vi "approach monitor.vi"() -> ()   [LabVIEW 2021]
uses:
  <userlib>/Nanonis Prog Interface V5/Nanonis Prog Interface.lvlib
panel:
  in  "Walker voltage (V)":dbl=220.0
  in  "stop":bool
  in  "Time between checks (ms)":i32=20000
  in  "Averages":i32=50
  in  "milliseconds to wait":u32=1000
  out "Delta":cluster{i32, sgl}[](graph)
  out "Capacitance":cluster{i32, sgl}[](graph)
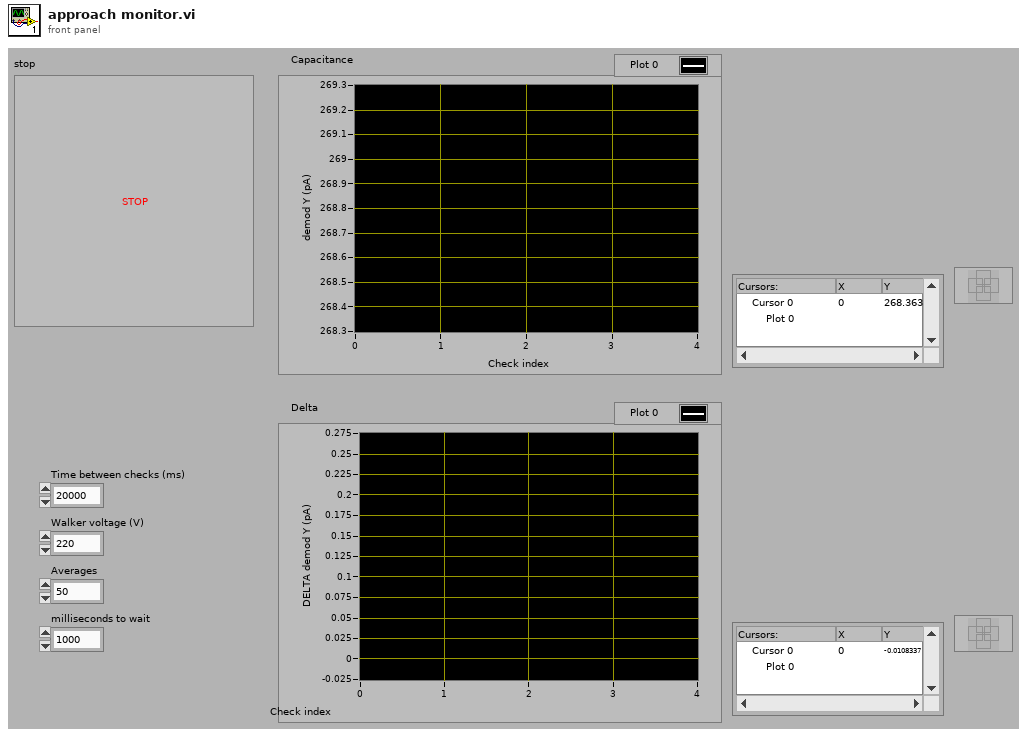
[diagram p1: front panel]
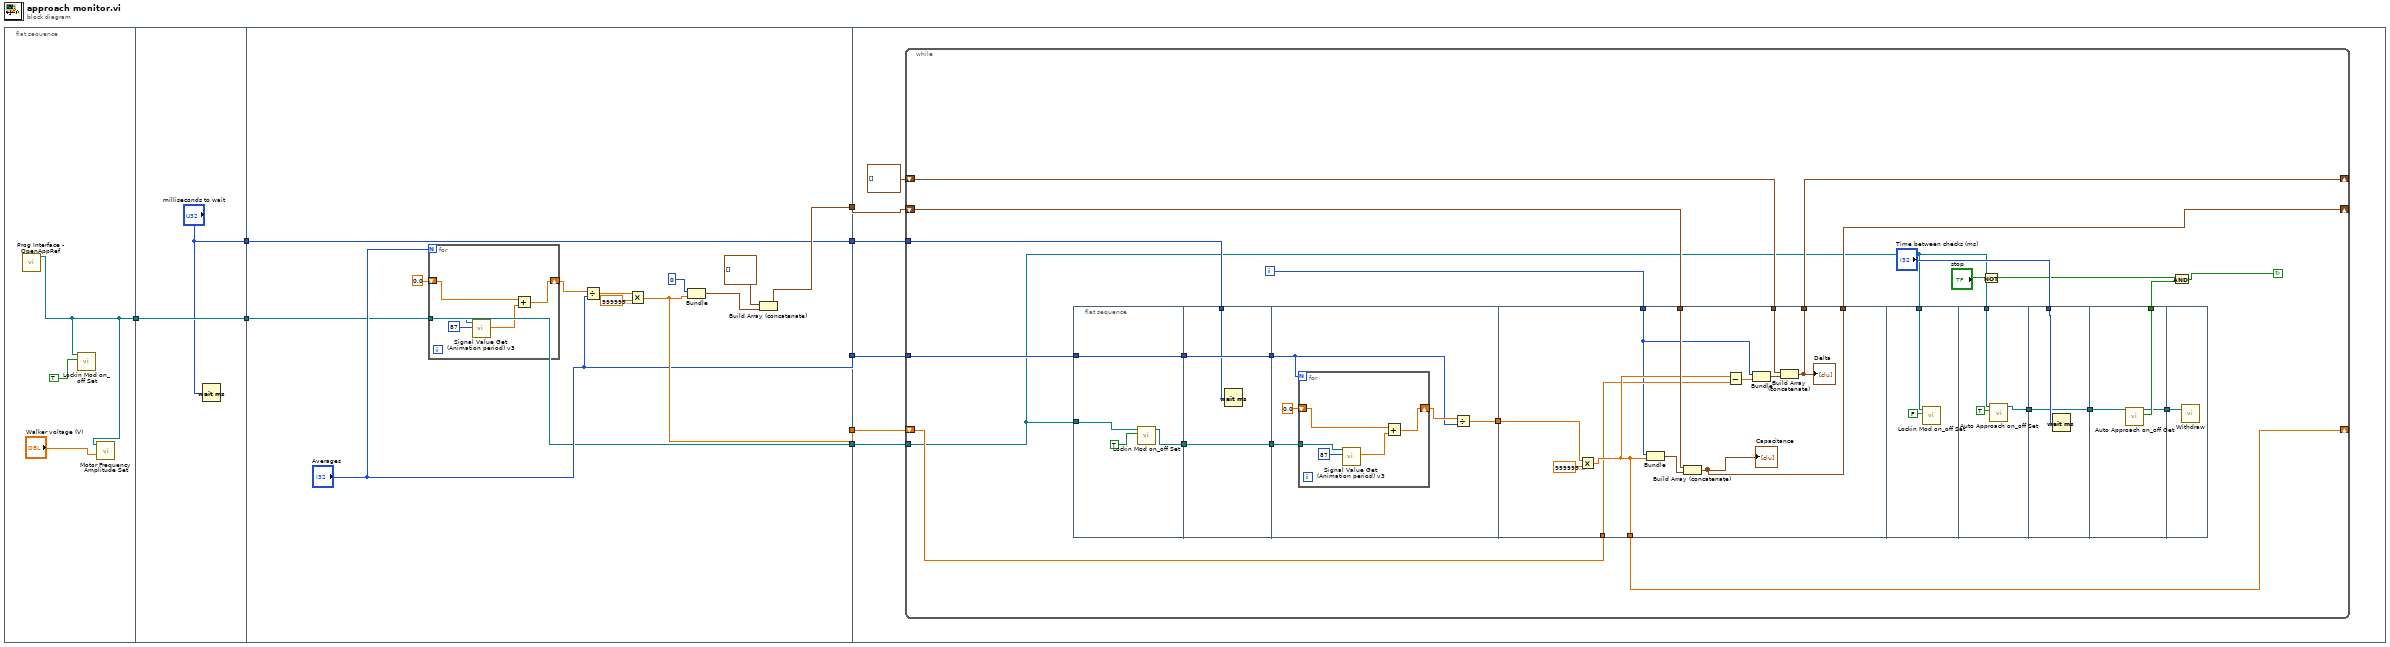
[diagram p0: block diagram]
diagram:
  n1 = flat-sequence {
    tunnel: [w9] -> w3
    tunnel: w3 -> [w13]
    tunnel: [w13] -> w2
    tunnel: ["milliseconds to wait"] -> w1
    tunnel: ["Averages"] -> w8
    tunnel: [w18] -> w7
    tunnel: [w21] -> w6
    tunnel: [w20] -> w5
    tunnel: w2 -> [w18]
    tunnel: [w17] -> w4
    tunnel: w1 -> [w17]
    tunnel: w8 -> [w36]
    tunnel: w7 -> [w35]
    tunnel: w6 -> [w34]
    tunnel: w5 -> [w33]
    tunnel: w4 -> [w31]
    frame #0 {
      n2 = call <userlib>:"Prog Interface - OpenAppRef.vi"() -> ("Application reference"=w9:refnum<vi>)  [unwired: 6 in, 1 out]
      n3 = call <userlib>:"Lockin Mod on_off Set.vi"("Lockin ON/OFF"=TRUE, "Application ref in"=w9) -> ()  [unwired: 8 in, 2 out]
      n4 = call <userlib>:"Motor Frequency Amplitude Set.vi"("Amplitude (V) (NaN=no change)"="Walker voltage (V)", "Application ref in"=w9) -> ()  [unwired: 8 in, 2 out]
    }
    frame #1 {
      n5 = Wait (ms)(milliseconds to wait="milliseconds to wait") -> ()  [unwired: 1 out]
    }
    frame #2 {
      n6 = for {
        N: "Averages" -> [_]
        shift-right: [w28] -> w24
        shift-left: sgl 0.0 ("Signal value") -> [w27]
        tunnel: w18 -> [w26]
        n7 = call <userlib>:"Signal Value Get (Animation period) v3.vi"("Signal index (0-127)"=i8 87, "Application ref in"=w26) -> ("Signal value"=w29:sgl)  [unwired: 6 in, 2 out]
        n8 = Add(x=w27, y=w29) -> (x+y=w28:sgl)
      }
      n9 = Divide(x=w24, y="Averages") -> (x/y=w25:sgl)
      n10 = Multiply(x=w25, y=sgl 1000000000000.0) -> (x*y=w20:sgl)
      n11 = Bundle(0, w20) -> (w15:cluster{i32, sgl})  [unwired: 1 in]
      n12 = Build Array (concatenate)(cluster{i32, sgl}[] [], w15) -> (w21:cluster{i32, sgl}[])
    }
    frame #3 {
      n13 = while {
        shift-right: [w58] -> _
        shift-left: w34 -> [w55]
        shift-right: [w57] -> _
        shift-left: cluster{i32, sgl}[] [] -> [w54]
        shift-right: [w53] -> _
        shift-left: w33 -> [w52]
        tunnel: w36 -> [w56]
        tunnel: w35 -> [w37]
        tunnel: w31 -> [w38]
        i -> [w43]
        stop <- w44 continue-if-true
        n14 = flat-sequence {
          tunnel: w37 -> [w62]
          tunnel: w56 -> [w63]
          tunnel: [w63] -> w42
          tunnel: [w61] -> w40
          tunnel: w42 -> [w66]
          tunnel: [w66] -> w41
          tunnel: w40 -> [w65]
          tunnel: [w65] -> w39
          tunnel: w38 -> [w64]
          tunnel: [w69] -> w59
          tunnel: w41 -> [w68]
          tunnel: w39 -> [w67]
          tunnel: w59 -> [w86]
          tunnel: [w84] -> w58
          tunnel: [w85] -> w57
          tunnel: w55 -> [w83]
          tunnel: w54 -> [w82]
          tunnel: [w81] -> w53
          tunnel: w52 -> [w80]
          tunnel: w43 -> [w79]
          tunnel: w37 -> [w89]
          tunnel: w37 -> [w92]
          tunnel: [w91] -> w49
          tunnel: "Time between checks (ms)" -> [w95]
          tunnel: [w94] -> w50
          tunnel: w49 -> [w94]
          tunnel: [w98] -> w45
          tunnel: w50 -> [w97]
          tunnel: [w96] -> w48
          tunnel: w48 -> [w99]
          frame #0 {
            n15 = call <userlib>:"Lockin Mod on_off Set.vi"("Lockin ON/OFF"=TRUE, "Application ref in"=w62) -> ("Application ref out"=w61:refnum<vi>)  [unwired: 8 in, 1 out]
          }
          frame #1 {
            n16 = Wait (ms)(milliseconds to wait=w64) -> ()  [unwired: 1 out]
          }
          frame #2 {
            n17 = for {
              N: w68 -> [_]
              shift-right: [w74] -> w70
              shift-left: sgl 0.0 ("Signal value") -> [w73]
              tunnel: w67 -> [w72]
              n18 = call <userlib>:"Signal Value Get (Animation period) v3.vi"("Signal index (0-127)"=i8 87, "Application ref in"=w72) -> ("Signal value"=w75:sgl)  [unwired: 6 in, 2 out]
              n19 = Add(x=w73, y=w75) -> (x+y=w74:sgl)
            }
            n20 = Divide(x=w70, y=w68) -> (x/y=w69:sgl)
          }
          frame #3 {
            n21 = Multiply(x=w86, y=sgl 1000000000000.0) -> (x*y=w81:sgl)
            n22 = Bundle(w79, w81) -> (w77:cluster{i32, sgl})  [unwired: 1 in]
            n23 = Build Array (concatenate)(w83, w77) -> (w84:cluster{i32, sgl}[])
            "Capacitance" <- w84
            n24 = Subtract(x=w81, y=w80) -> (x-y=w88:sgl)
            n25 = Bundle(w79, w88) -> (w78:cluster{i32, sgl})  [unwired: 1 in]
            n26 = Build Array (concatenate)(w82, w78) -> (w85:cluster{i32, sgl}[])
            "Delta" <- w85
          }
          frame #4 {
            n27 = call <userlib>:"Lockin Mod on_off Set.vi"("Lockin ON/OFF"=FALSE, "Application ref in"=w89) -> ()  [unwired: 8 in, 2 out]
          }
          frame #5 {
            n28 = call <userlib>:"Auto Approach on_off Set.vi"("Auto approach start/stop (F)"=TRUE, "Application ref in"=w92) -> ("Application ref out"=w91:refnum<vi>)  [unwired: 6 in, 1 out]
          }
          frame #6 {
            n29 = Wait (ms)(milliseconds to wait=w95) -> ()  [unwired: 1 out]
          }
          frame #7 {
            n30 = call <userlib>:"Auto Approach on_off Get.vi"("Application ref in"=w97) -> ("Auto approach on/off status"=w98:bool, "Application ref out"=w96:refnum<vi>)  [unwired: 6 in, 1 out]
          }
          frame #8 {
            n31 = call <userlib>:"Withdraw.vi"("Application ref in"=w99) -> ()  [unwired: 9 in, 2 out]
          }
        }
        n32 = Not(x="stop") -> (.not. x?=w46:bool)
        n33 = And(x=w46, y=w45) -> (x .and. y?=w44:bool)
      }
    }
  }
